vi "Get Item.vi"(8 "error in (no error)":errorcluster, 11 "ScrollingList in":refnum<class "ScrollingList.lvclass">) -> (0 "error out":errorcluster, 3 "ScrollingList (dup)":refnum<class "ScrollingList.lvclass">)   [LabVIEW 2020, in "ScrollingList.lvclass"]
uses:
  ScrollingList.lvclass
  ScrollingList.lvclass/ScrollingList.ctl
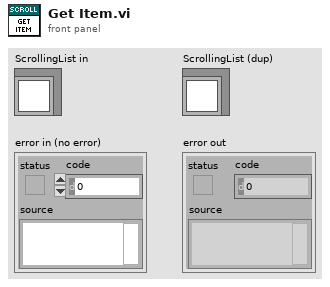
[diagram p1: front panel]
types:
  T1 = typedef "ScrollingList.lvclass/State Data.ctl" = cluster{"Timeout":i32, "Time":timestamp, "Y":i32, "Origin:Top":i16, "Rate":dbl, "ListItems":string[], "Item Height":i32, "Max Height":i32}
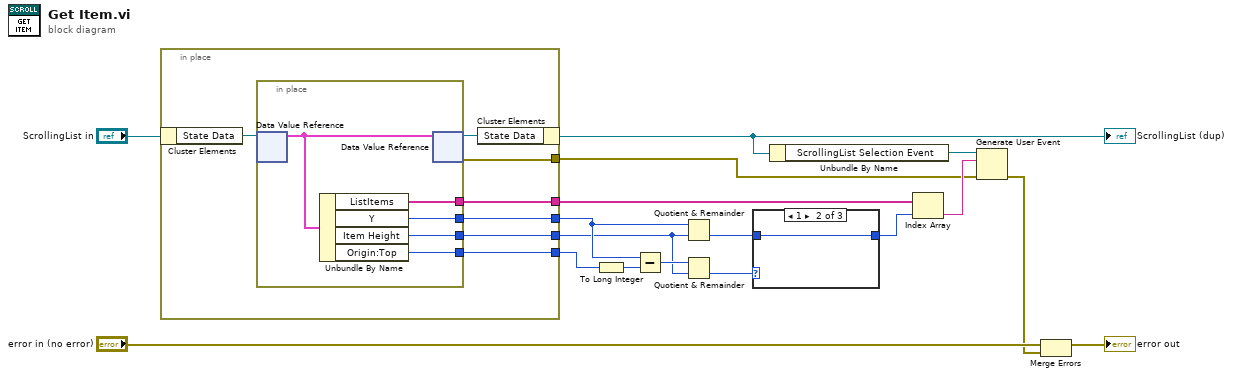
[diagram p0: block diagram]
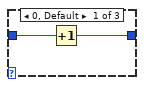
[diagram p2: hidden frame]
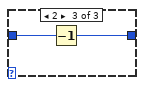
[diagram p3: hidden frame]
diagram:
  n1 = in-place {
    in-place-border: [w23] -> w9
    in-place-border: [w21] -> w12
    in-place-border: [w20] -> w11
    in-place-border: [w19] -> w10
    in-place-border: [w18] -> w6
    n2 = in-place-cluster #1("ScrollingList in") -> ("State Data"=w24:refnum<data-value>)
    n3 = in-place {
      in-place-border: [w28] -> w23
      in-place-border: [w27] -> w21
      in-place-border: [w26] -> w20
      in-place-border: [w25] -> w19
      n4 = in-place-dvr #2(w24) -> (w29:T1)  [unwired: 1 out]
      n5 = Unbundle By Name(w29) -> ("ListItems"=w28:string[], "Y"=w27:i32, "Item Height"=w26:i32, "Origin:Top"=w25:i16)
      n6 = in-place-dvr #2(w29) -> (w22:refnum<data-value>, w18:errorcluster)
    }
    n7 = in-place-cluster #1("State Data"=w22) -> (w1:refnum<class "ScrollingList.lvclass">)
  }
  "ScrollingList (dup)" <- w1
  n8 = To Long Integer(number=w10) -> (32bit integer=w13:i32)
  n9 = Subtract(x=w12, y=w13) -> (x-y=w14:i32)
  n10 = Quotient & Remainder(x=w12, y=w11) -> (floor(x/y)=w16:i32)  [unwired: 1 out]
  n11 = Quotient & Remainder(x=w14, y=w11) -> (floor(x/y)=w15:i32)  [unwired: 1 out]
  n12 = case shown="1" w15 {
    tunnel: [w30 w32 w33] -> w2
    tunnel: w16 -> [w31 w32 w34]
    frame 0, Default {
      n13 = Increment(x=w31) -> (x+1=w30:i32)
    }
    frame 1 {
    }
    frame 2 {
      n14 = Decrement(x=w34) -> (x-1=w33:i32)
    }
  }
  n15 = Unbundle By Name(w1) -> ("ScrollingList Selection Event"=w8:refnum<user-event>)
  n16 = Index Array(array=w9, index=w2) -> (element=w7:string)
  n17 = Generate User Event(user event=w8, event data cluster=w7, error in=w6) -> (error out=w3:errorcluster)  [unwired: 1 in, 1 out]
  n18 = Merge Errors("error in (no error)", w3) -> (→"error out":errorcluster)
